vi "Translator.Global.vi"() -> ()   [LabVIEW 2019, in "Tools.lvlib"]
uses:
  Tools.lvlib
panel:
  in  "tab":enum32{"General", "more..."}(tab)
  out "Translations.Event":string[](array[string])
  out "Translations.Status":string[](array[string])
  out "Translations.Level":string[](array[string])
  out "Translations.ExitAction":string[](array[string])
  out "Translations.Months":string[](array[string])
  out "Translations.Vision.ImgSelect":string[](array[string])
  out "Translations.Menu":string[](array[string])
  out "Translations.Items":string[](array[string])
  in  "FilePath":path
  out "Font":string
  in  "TranslatedVIs":string[](array[string])=["MainGui.vi", "Translator.MainGui.vi", "Translator.SelectLanguageGui.vi", "User.LoginGui.vi", "User.SettingsGui.vi", "EventLog.Gui.vi", "ErrorHandling.Gui.vi", "Wait.Gui.vi", "AboutGui.vi", "InfoGui.vi", "ExitGui.vi", "Vision.Gui.vi"]
  in  "Applicaiton INI file":path
  out "Languages":string[](array[string])
  out "Flag":picture
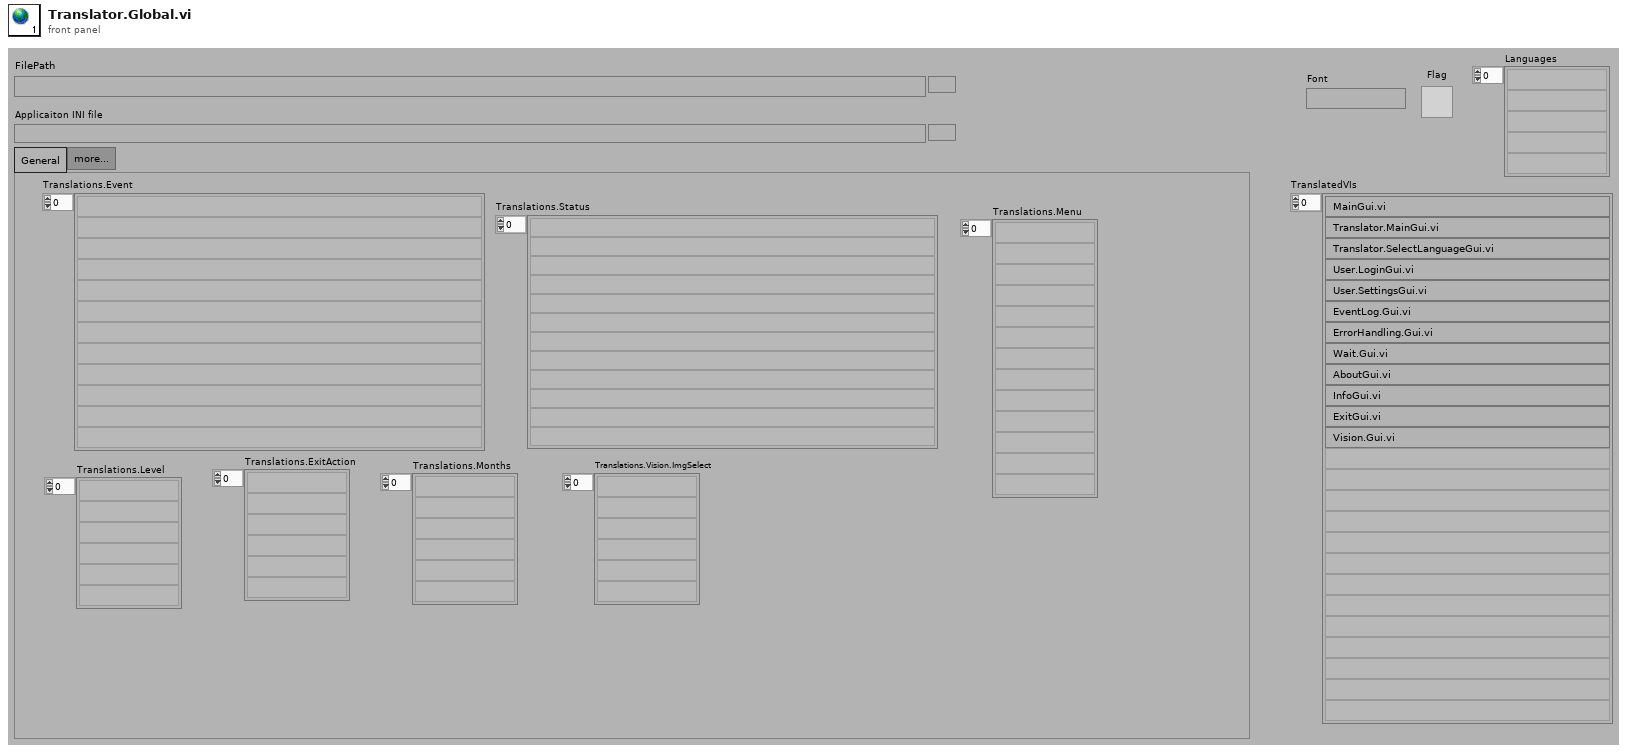
[diagram p1: front panel]
diagram:
